vi "BinToDec.vi"(2 "error in":errorcluster, 3 "Number Format (bin)":enum16{"binary", "hex", "octal"}(ring), 4 "Number String (0010)":string="0010") -> (0 "error out":errorcluster, 1 "Converted number (decimal)":i32=2)   [LabVIEW 2022 SP3]
doc: "This VI will convert a binary, hexadecimal, or octal number into a decimal value. The input value is a string, and can have any number of leading zeroes."
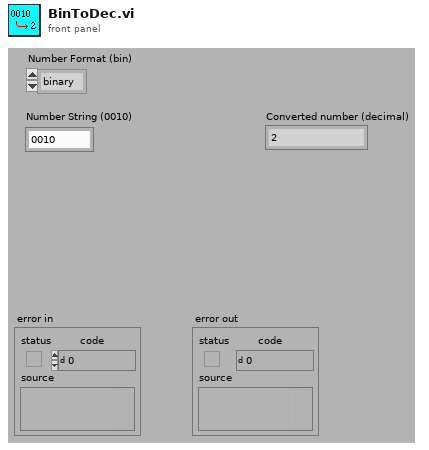
[diagram p1: front panel]
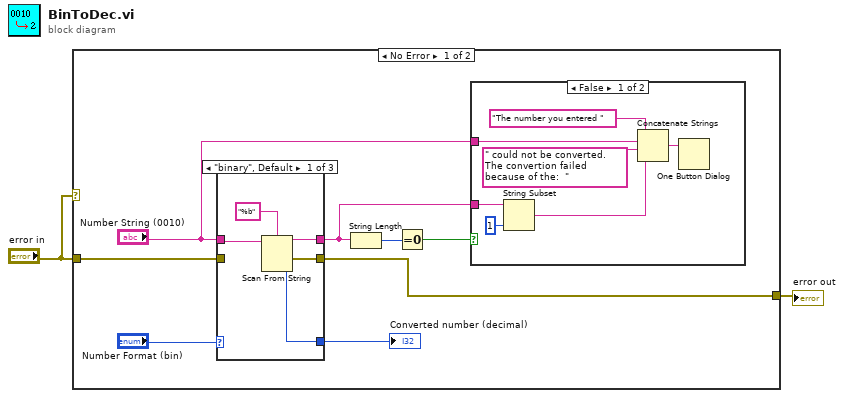
[diagram p0: block diagram]
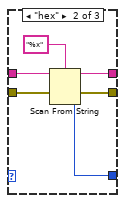
[diagram p3: hidden frame]
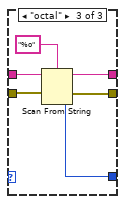
[diagram p4: hidden frame]
diagram:
  n1 = case shown="No Error" "error in" {
    tunnel: "error in" -> [w8 w35]
    tunnel: [w3 w35] -> w1
    frame No Error {
      n2 = case shown="\"binary\", Default" "Number Format (bin)" {
        tunnel: "Number String (0010)" -> [w22 w28 w34]
        tunnel: [w20 w26 w30] -> w9
        tunnel: w8 -> [_ w25 w33]
        tunnel: [w19 w24 w31] -> w3
        tunnel: [w18 w23 w29] -> w5
        frame "binary", Default {
          n3 = Scan From String(format string="%b" ("Format String"), input string=w22) -> (remaining string=w18:string, error out=w19:errorcluster, output 1=w20:i32)  [unwired: 2 in, 2 out]
        }
        frame "hex" {
          n4 = Scan From String(format string="%x" ("Format String"), input string=w28, error in=w25) -> (remaining string=w23:string, error out=w24:errorcluster, output 1=w26:u32)  [unwired: 1 in, 2 out]
        }
        frame "octal" {
          n5 = Scan From String(format string="%o" ("Format String"), input string=w34, error in=w33) -> (remaining string=w29:string, error out=w31:errorcluster, output 1=w30:i32)  [unwired: 1 in, 2 out]
        }
      }
      "Converted number (decimal)" <- w9
      n6 = String Length(string=w5) -> (length=w7:i32)
      n7 = Equal To 0?(x=w7) -> (x = 0?=w6:bool)
      n8 = case shown="False" w6 {
        tunnel: w5 -> [w16 _]
        tunnel: "Number String (0010)" -> [w15 _]
        frame False {
          n9 = String Subset(string=w16, length (rest)=1 ("length (rest)")) -> (substring=w12:string)  [unwired: 1 out]
          n10 = Concatenate Strings("The number you entered ", w15, " could not be converted.  The convertion failed because of the:  " ("Substring"), w12) -> (w11:string)
          n11 = One Button Dialog(message=w11) -> ()  [unwired: 2 out]
        }
        frame True {
          # "no error in the conversion"
        }
      }
    }
    frame Error {
      # "error in = true"
    }
  }
  "error out" <- w1
